vi "Read Sensor Data.vi"(3 "error in (no error)":errorcluster, 5 "VISA resource name":refnum<visa-resource-name>) -> (0 "error out":errorcluster, 1 "Data out":T1, 2 "VISA resource name out":refnum<visa-resource-name>)   [LabVIEW 2021, in "IMU Acquisition.lvlib"]
uses:
  IMU Acquisition.lvlib
  IMU TimeDataStruct.ctl
panel:
  in  "String":string="%d_%m_%Y_%H_%M_%S_%4u"
  out "date/time string":string
  out "return count":u32=56
  out "read buffer":string="0.85\t-24.90\t-990.72\t0.84\t-0.23\t0.46\t-35.25\t3.30\t-50.55\r\n"
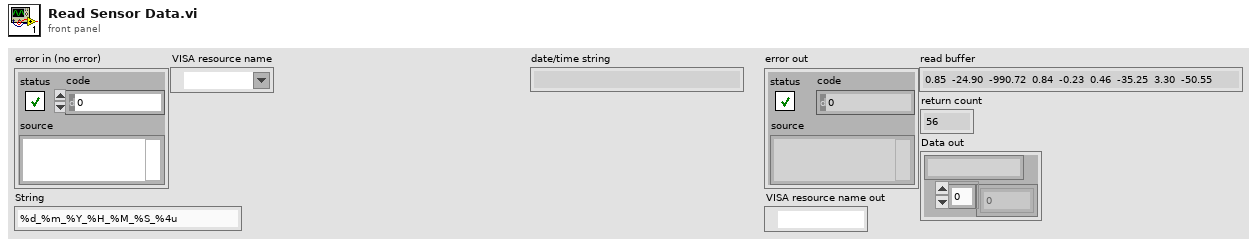
[diagram p1: front panel]
types:
  T1 = typedef "IMU TimeDataStruct.ctl" = cluster{string, dbl[]}
  T2 = cluster{"date/time string":string, "array type (2D Dbl)":dbl[]}
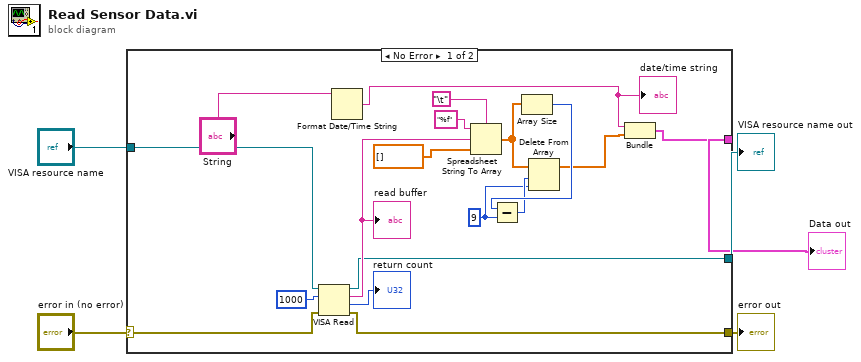
[diagram p0: block diagram]
diagram:
  n1 = case shown="No Error" "error in (no error)" {
    selector: "error in (no error)" -> [w18 w25]
    tunnel: [w17 w25] -> w4
    tunnel: "VISA resource name" -> [w15 w24]
    tunnel: [w14 w24] -> w2
    tunnel: [w7 _] -> w1
    frame No Error {
      w10 = 9 ("y")
      n2 = VISA Read(VISA resource name=w15, byte count=u32 1000, error in (no error)=w18) -> (VISA resource name out=w14:refnum<visa-resource-name>, read buffer=w22:string, return count=→"return count":u32, error out=w17:errorcluster)
      "read buffer" <- w22
      n3 = Format Date/Time String(time format string (%c)="String") -> (date/time string=w6:string)  [unwired: 2 in]
      "date/time string" <- w6
      n4 = Spreadsheet String To Array(delimiter (Tab)="\t", format string="%f", spreadsheet string=w22, array type (2D Dbl)=dbl[] []) -> (array=w13:dbl[])
      n5 = Array Size(array=w13) -> (size(s)=w12:i32)
      n6 = Subtract(x=w12, y=w10) -> (x-y=w11:i32)
      n7 = Delete From Array(array=w13, length=w11, index=w10) -> (array with subset deleted=w8:dbl[])  [unwired: 1 out]
      n8 = Bundle("date/time string"=w6, "array type (2D Dbl)"=w8) -> (w7:T2)  [unwired: 1 in]
    }
    frame Error {
    }
  }
  "error out" <- w4
  "VISA resource name out" <- w2
  "Data out" <- w1
